vi "SH_generateShapelets_Pruning.vi"(5 "MaxLength (in %)":dbl(slide) min=0.0 max=1.0 step=0.05 scale=0.0..1.0, 7 "MinLength (in %)":dbl(slide) min=0.0 max=1.0 step=0.05 scale=0.0..1.0, 8 "error in (no error)":errorcluster, 9 "Progress":refnum<vi>, 10 "Shapelets Queue":refnum<queue>, 11 "ShapeletClass in":refnum<class "Shapelets Search Brute Force.lvclass">) -> (0 "error out":errorcluster, 2 "Total Number of Shapelets":i32, 3 "ShapeletClass out":refnum<class "Shapelets Search Brute Force.lvclass">)   [LabVIEW 2016, in "Shapelets Search (Brute Force).lvlib" / "Shapelets Search Brute Force.lvclass"]
uses:
  Shapelets Search Brute Force.lvclass
  SH_Shapelet.ctl
  Shapelets Search Brute Force.lvclass/Shapelets Search Brute Force.ctl
  <vilib>/Analysis/baseanly.llb/Normalize Vector.vi
  Shapelets Search (Brute Force).lvlib
  5. Features Optimization/_Optimal Frequency Bands Search/Optimal Frequency Bands Search.lvlib
  <vilib>/Analysis/NI_AALBase.lvlib
panel:
  # "This VI is a part of BCI Design library, http://www.ru-bci.org \nCopyright © 2020, Sotnikov Peter, All rights reserved. License: CC BY-NC 4.0"
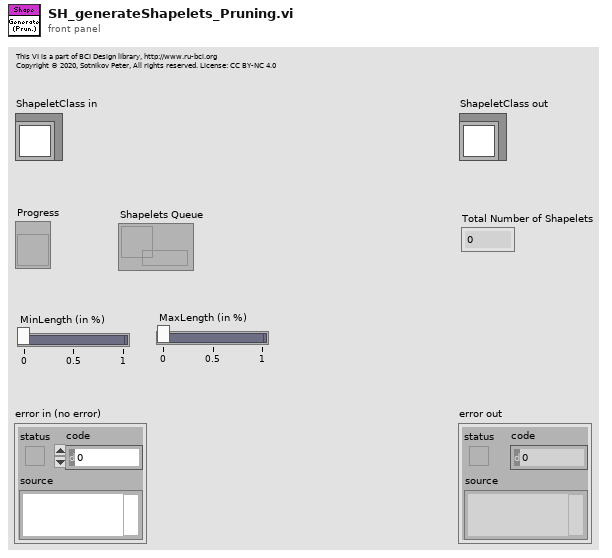
[diagram p1: front panel]
types:
  T1 = typedef "Shapelets Search (Brute Force).lvlib/SH_Shapelet.ctl" = cluster{"TrialIndex":i32, "Shift (in samples)":i32, "Length (in samples)":i32, "Distances":dbl[], "ClassIndecies":i32[], "Fitness":dbl, "Split Point":dbl}
  T2 = cluster{"ClassLabel":string, "FeatureVector":dbl[][]}[]
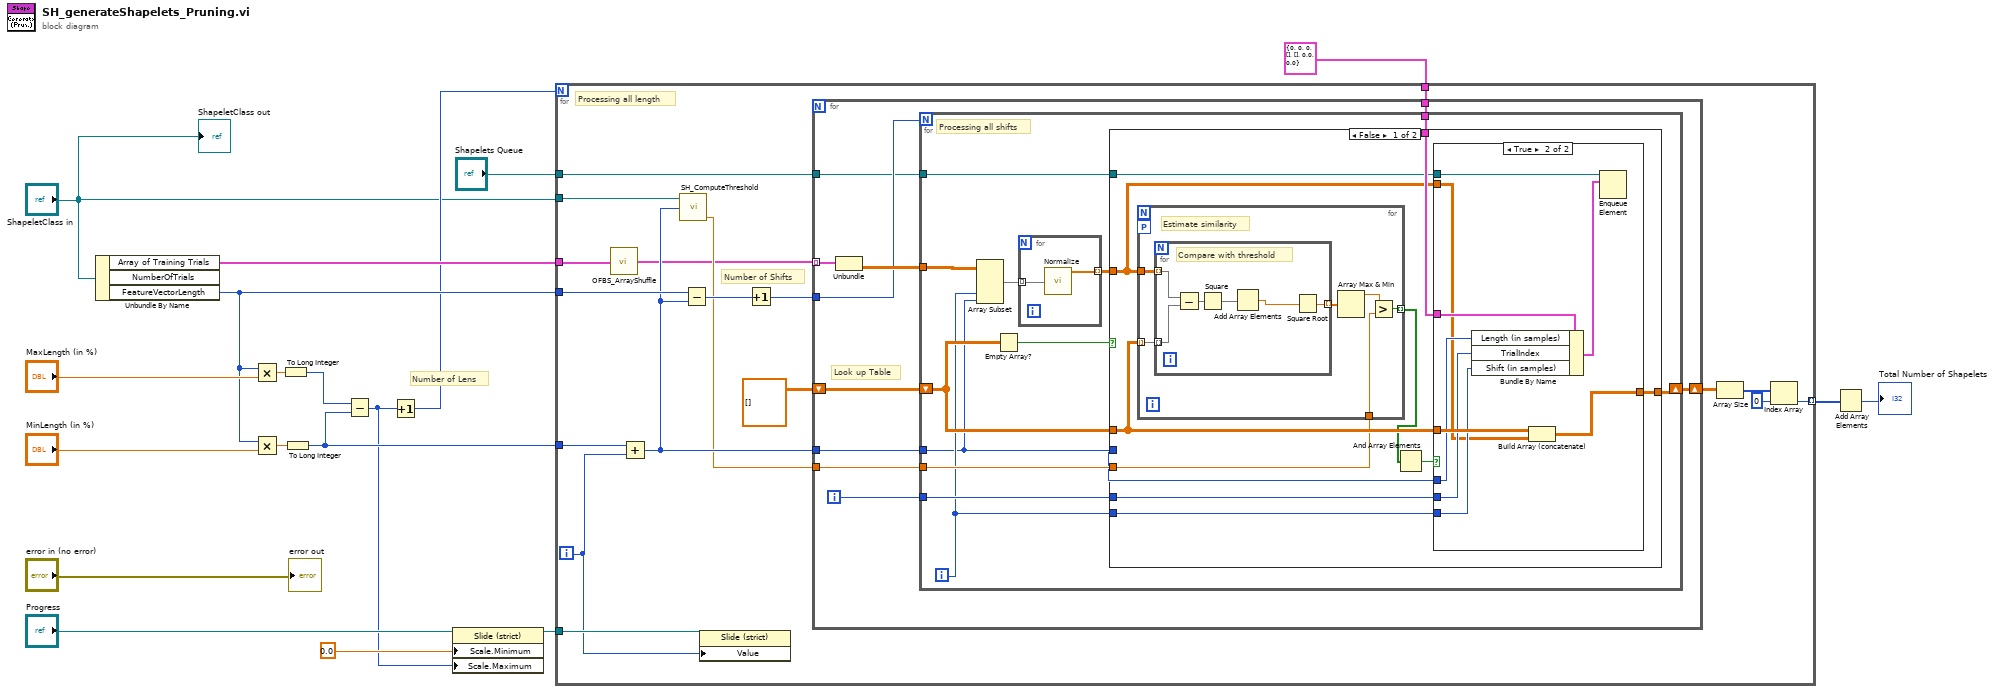
[diagram p0: block diagram]
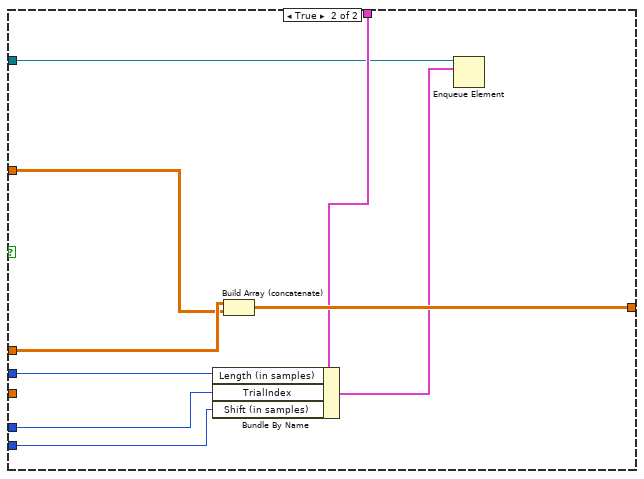
[diagram p3: hidden frame]
diagram:
  # "Number of Lens"
  n1 = Unbundle By Name("ShapeletClass in") -> ("Array of Training Trials"=w11:T2, "FeatureVectorLength"=w9:i32)  [unwired: 1 out]
  n2 = Multiply(x=w9, y="MaxLength (in %)") -> (x*y=w14:dbl)
  n3 = Multiply(x=w9, y="MinLength (in %)") -> (x*y=w13:dbl)
  n4 = To Long Integer(number=w14) -> (32bit integer=w12:i32)
  n5 = To Long Integer(number=w13) -> (32bit integer=w10:i32)
  n6 = Subtract(x=w12, y=w10) -> (x-y=w1:i32)
  n7 = Increment(x=w1) -> (x+1=w5:i32)
  n8 = property class="Slide (strict)"(reference="Progress", "Scale.Minimum"=0.0 ("Data Entry Limits:Minimum"), "Scale.Maximum"=w1) -> (reference out=w6:refnum<vi>)  [unwired: 1 in, 1 out]
  n9 = for {
    N: w5 -> [_]
    tunnel: w11 -> [w21]
    tunnel: w10 -> [w37]
    tunnel: w9 -> [w36]
    tunnel: [w28] -> w8 mode=indexing
    tunnel: w6 -> [w27]
    tunnel: T1 {"TrialIndex"=0, "Shift (in samples)"=0, "Length (in samples)"=0, "Distances"=[], "ClassIndecies"=[], "Fitness"=0.0, "Split Point"=0.0} ("Shapelet") -> [w25]
    tunnel: "ShapeletClass in" -> [w24]
    tunnel: "Shapelets Queue" -> [w23]
    i -> [w26]
    # "Number of Shifts"
    # "Processing all length"
    n10 = call "OFBS_ArrayShuffle.vi"("Array in"=w21) -> ("Array out"=w20:cluster{"ClassLabel":string, "Trial":dbl[][]}[])
    n11 = Add(x=w37, y=w26) -> (x+y=w34:i32)
    n12 = call "SH_ComputeThreshold.vi"("Shapelet Length"=w34, "ShapeletClass in"=w24) -> ("percentile"=w22:dbl)  [unwired: 2 in, 1 out]
    n13 = Subtract(x=w36, y=w34) -> (x-y=w35:i32)
    n14 = property class="Slide (strict)"(reference=w27, "Value"=w26) -> ()  [unwired: 1 in, 2 out]
    n15 = Increment(x=w35) -> (x+1=w32:i32)
    n16 = for {
      tunnel: w22 -> [w47]
      tunnel: w34 -> [w46]
      tunnel: w20 -> [w45] mode=indexing
      shift-right: [w41] -> w31
      shift-left: dbl[][][] [] -> [w42]
      tunnel: w32 -> [w43]
      tunnel: w25 -> [w39]
      tunnel: w23 -> [w38]
      i -> [w40]
      # "Look up Table"
      n17 = Unbundle(w45) -> ("Trial"=w44:dbl[][])  [unwired: 1 out]
      n18 = for {
        N: w43 -> [_]
        tunnel: w47 -> [w55]
        tunnel: w46 -> [w50]
        tunnel: w44 -> [w59]
        shift-right: [w56] -> w41
        shift-left: w42 -> [w57]
        tunnel: w40 -> [w54]
        tunnel: w39 -> [w53]
        tunnel: w38 -> [w52]
        i -> [w51]
        # "Processing all shifts"
        n19 = Array Subset(array=w59, index (col)=w51, length (col)=w50) -> (w49:dbl[][])  [unwired: 2 in]
        n20 = Empty Array?(array=w57) -> (empty?=w58:bool)
        n21 = for {
          tunnel: w49 -> [w61] mode=indexing
          tunnel: [w60] -> w48 mode=indexing
          n22 = call-poly <vilib>:"Normalize.vi"("Vector"=w61) -> ("Normalized Vector"=w60:dbl[])  [unwired: 1 in, 3 out]
        }
        n23 = case shown="False" w58 {
          tunnel: w57 -> [w67 w103]
          tunnel: [w72 w102] -> w56
          tunnel: w55 -> [w65 _]
          tunnel: w50 -> [w66 w100]
          tunnel: w54 -> [w71 w99]
          tunnel: w51 -> [w70 w98]
          tunnel: w53 -> [w69 w101]
          tunnel: w52 -> [w68 w97]
          tunnel: w48 -> [w62 w95]
          frame False {
            n24 = for {
              tunnel: w67 -> [w78] mode=indexing
              tunnel: w62 -> [w77]
              tunnel: w65 -> [w76]
              tunnel: [w75] -> w63 mode=indexing
              workers-P: _ -> [_]
              # "Estimate similarity"
              n25 = for {
                tunnel: w78 -> [w81] mode=indexing
                tunnel: w77 -> [w82] mode=indexing
                tunnel: [w80] -> w74 mode=indexing
                # "Compare with threshold"
                n26 = Subtract(x=w82, y=w81) -> (x-y=w84:dbl[])
                n27 = Square(x=w84) -> (x^2=w83:dbl[])
                n28 = Add Array Elements(numeric array=w83) -> (sum=w79:dbl)
                n29 = Square Root(x=w79) -> (sqrt(x)=w80:dbl)
              }
              n30 = Array Max & Min(array=w74) -> (max value=w73:dbl)  [unwired: 3 out]
              n31 = Greater?(x=w73, y=w76) -> (0:w75:bool)
            }
            n32 = And Array Elements(Boolean array=w63) -> (logical AND=w64:bool)
            n33 = case shown="True" w64 {
              tunnel: w67 -> [w85 w94]
              tunnel: [w85 w93] -> w72
              tunnel: w66 -> [_ w91]
              tunnel: w71 -> [_ w90]
              tunnel: w70 -> [_ w89]
              tunnel: w69 -> [_ w92]
              tunnel: w68 -> [_ w88]
              tunnel: w62 -> [_ w86]
              frame False {
              }
              frame True {
                n34 = Bundle By Name(cluster=w92, "Length (in samples)"=w91, "TrialIndex"=w90, "Shift (in samples)"=w89) -> (w87:T1)
                n35 = Build Array (concatenate)(w94, w86) -> (w93:dbl[][][])
                n36 = Enqueue Element(queue=w88, element=w87) -> ()  [unwired: 2 in, 3 out]
              }
            }
          }
          frame True {
            n37 = Bundle By Name(cluster=w101, "Length (in samples)"=w100, "TrialIndex"=w99, "Shift (in samples)"=w98) -> (w96:T1)
            n38 = Build Array (concatenate)(w103, w95) -> (w102:dbl[][][])
            n39 = Enqueue Element(queue=w97, element=w96) -> ()  [unwired: 2 in, 3 out]
          }
        }
      }
    }
    n40 = Array Size(array=w31) -> (size(s)=w30:i32[])
    n41 = Index Array(array=w30, index=0) -> (element=w28:i32)
  }
  n42 = Add Array Elements(numeric array=w8) -> (sum=→"Total Number of Shapelets":i32)
  "error out" <- "error in (no error)"
  "ShapeletClass out" <- "ShapeletClass in"
